vi "simple_01.vi"() -> ()   [LabVIEW 2014]
uses:
  builds/LVTables/SQLite Packed/SQLite3LV.lvlibp/Cursor Class/property binding/column I32.vi
  builds/LVTables/SQLite Packed/SQLite3LV.lvlibp/Cursor Class/Fetch N - String.vi
  builds/LVTables/SQLite Packed/SQLite3LV.lvlibp/SQLite3 Class/sqlite3.lvclass
  builds/LVTables/SQLite Packed/SQLite3LV.lvlibp/Cursor Class/cursor.lvclass
panel:
  out "Persons":string[][](array[string])
  out "result":i32
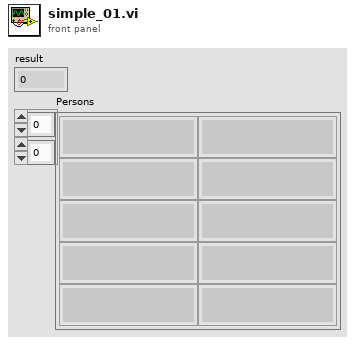
[diagram p1: front panel]
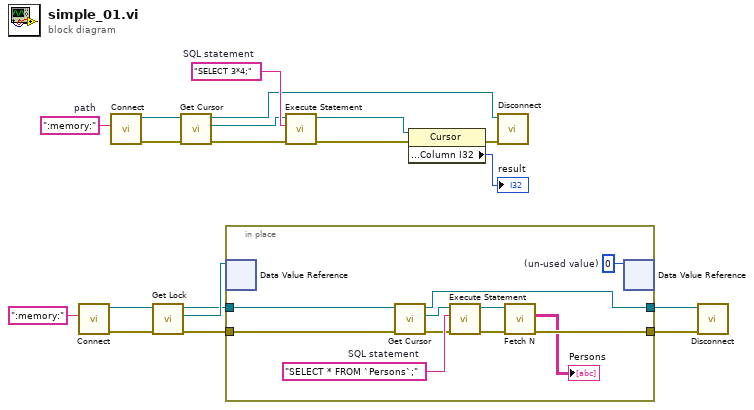
[diagram p0: block diagram]
diagram:
  w15 = "SELECT 3*4;"  # SQL statement
  w17 = ":memory:"  # path
  n1 = call "Connect.vi"("path"=":memory:") -> ("error out"=w6:errorcluster, "SQLite3LV Connection out"=w3:refnum<class "sqlite3.lvclass">)  [unwired: 9 in]
  n2 = call "Connect.vi"("path"=w17) -> ("error out"=w18:errorcluster, "SQLite3LV Connection out"=w19:refnum<class "sqlite3.lvclass">)  [unwired: 9 in]
  n3 = call "Get Lock.vi"("error in (no error)"=w6, "SQLite3LV Connection in"=w3) -> ("error out"=w4:errorcluster, "sqlite lock"=w5:refnum<data-value>, "SQLite3LV Connection out"=w2:refnum<class "sqlite3.lvclass">)  [unwired: 7 in]
  n4 = call "Get Cursor.vi"("error in (no error)"=w18, "SQLite3LV Connection in"=w19) -> ("error out"=w16:errorcluster, "SQLite3LV Cursor"=w1:refnum<class "cursor.lvclass">, "SQLite3LV Connection out"=w10:refnum<class "sqlite3.lvclass">)  [unwired: 7 in]
  n5 = in-place "In Place Element Structure" {
    in-place-border: [w30] -> w9
    in-place-border: [w22] -> w8
    in-place-border: w4 -> [w26]
    in-place-border: w2 -> [w25]
    w20 = 0  # (un-used value)
    w29 = "SELECT * FROM `Persons`;"  # SQL statement
    n6 = in-place-dvr #1(w5) -> ()  [unwired: 2 out]
    n7 = call "Get Cursor.vi"("error in (no error)"=w26, "SQLite3LV Connection in"=w25) -> ("error out"=w28:errorcluster, "SQLite3LV Cursor"=w27:refnum<class "cursor.lvclass">, "SQLite3LV Connection out"=w30:refnum<class "sqlite3.lvclass">)  [unwired: 7 in]
    n8 = call "Execute Statement.vi"("error in (no error)"=w28, "SQL statement"=w29, "SQLite3LV Cursor in"=w27) -> ("error out"=w23:errorcluster, "SQLite3LV Cursor out"=w24:refnum<class "cursor.lvclass">)  [unwired: 7 in]
    n9 = call-poly "Fetch N.vi"("error in (no error)"=w23, "SQLite3LV Cursor in"=w24) -> ("error out"=w22:errorcluster, "result"=→"Persons":string[][])  [unwired: 6 in, 2 out]
    n10 = in-place-dvr #1(w20) -> ()  [unwired: 2 out]
  }
  n11 = call "Execute Statement.vi"("error in (no error)"=w16, "SQL statement"=w15, "SQLite3LV Cursor in"=w1) -> ("error out"=w13:errorcluster, "SQLite3LV Cursor out"=w14:refnum<class "cursor.lvclass">)  [unwired: 7 in]
  n12 = property class="Cursor"(reference=w14, error in=w13) -> (error out=w11:errorcluster, "property binding:Column I32"=→"result":i32)  [unwired: 1 out]
  n13 = call "Disconnect.vi"("error in (no error)"=w11, "SQLite3LV Connection in"=w10) -> ()  [unwired: 9 in, 1 out]
  n14 = call "Disconnect.vi"("error in (no error)"=w8, "SQLite3LV Connection in"=w9) -> ()  [unwired: 9 in, 1 out]
